vi "HMI object.vi"(4 "HMI VI path":path, 6 "Subpanel ref":refnum<vi>, 8 "error in":errorcluster, 9 "HMI cluster":T2={"Elapsed time in current state"=0.0, "smooth interval (s)"=0.0, "Process State"=1, "Current Control settings"=[]} {"Current Control settings"."fractional duty" format="%#_3g"; "smooth interval (s)" format="%.3f"; "Elapsed time in current state" format="%.2f"}, 11 "command":T4) -> (0 "error out":errorcluster, 1 "HMI Failure":bool, 3 "HMI VI ref out":T3)   [LabVIEW 2012]
uses:
  HMI command.ctl
  HMI VI type.ctl
  switch and fraction.ctl
  DAQ configuration/Sensor buffer command.ctl
  logic buffer cmd.ctl
panel:
  in  "Control names":string[](array[string])=["Current Control settings", "Sensor Data smoothed", "Set Points", "Elapsed time in current state", "Process State"]
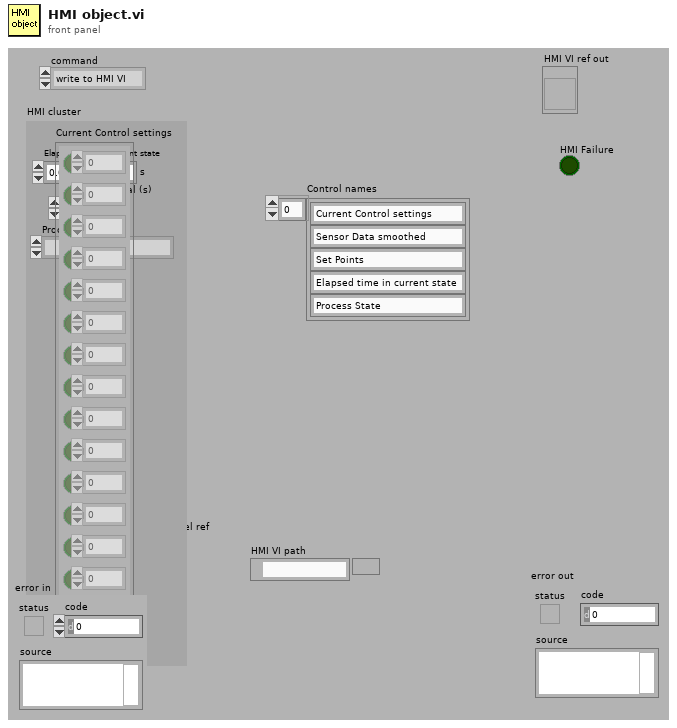
[diagram p1: front panel]
types:
  T1 = typedef "switch and fraction.ctl" = cluster{"switch":bool, "fractional duty":dbl}[]
  T2 = cluster{"Elapsed time in current state":dbl, "smooth interval (s)":sgl, "Process State":u16, "Current Control settings":T1}
  T3 = typedef "HMI VI type.ctl" = refnum<vi>
  T4 = typedef "HMI command.ctl" = enum16{"write to HMI VI", "Disconnect HMI VI", "Connect HMI VI", "Load Subpanel"}
  T5 = typedef "logic buffer cmd.ctl" = enum16{"read", "write ouput settings", "write rules", "write setpoints", "write output descriptions", "write all", "calculate setpoints", "save", "open", "Load all setpoint code", "Load one setpoint code", "Configure one setpoint code"}
  T6 = typedef "Sensor buffer command.ctl" = enum16{"read average", "read recent", "read all", "write", "configure", "clear"}
  T7 = typedef "variable setpoint.ctl" = cluster{"name":string, "unit":string, "value":dbl, "Type":enum16{"Constant", "Variable"}, "variable":cluster{"selected sensors":i32[], "selected set points":i32[], "VI":path, "Data average interval":T8, "code ref":T9}}
  T8 = typedef "data ave interval.ctl" = dbl
  T9 = typedef "type specifier for control code.ctl" = refnum<vi>
  T10 = typedef "Sensor data.ctl" = cluster{" Sensor array":T11[], "Time":dbl}
  T11 = typedef "sensor cluster.ctl" = cluster{"voltage":sgl, "scaled":sgl, "units":string, "Out of Range":bool}
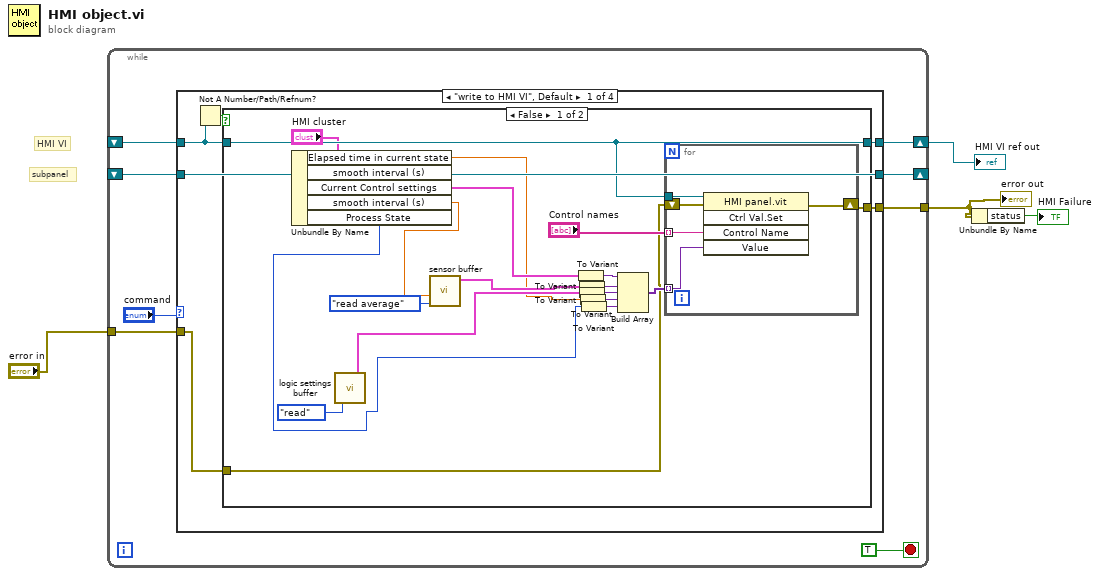
[diagram p0: block diagram]
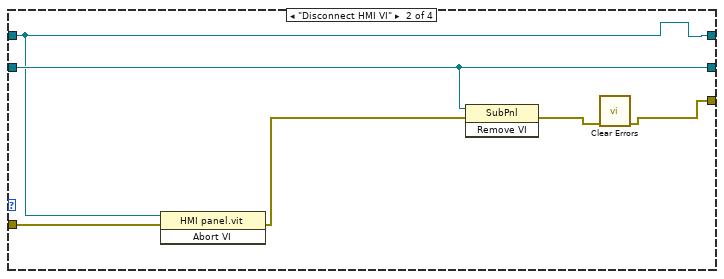
[diagram p3: hidden frame]
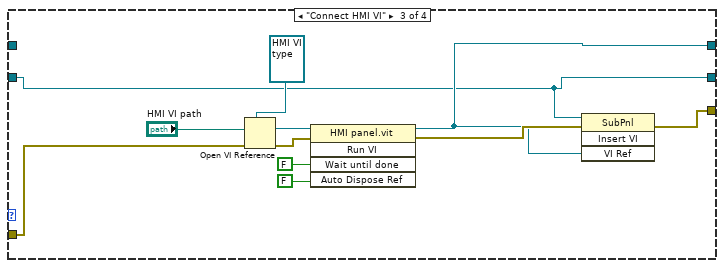
[diagram p4: hidden frame]
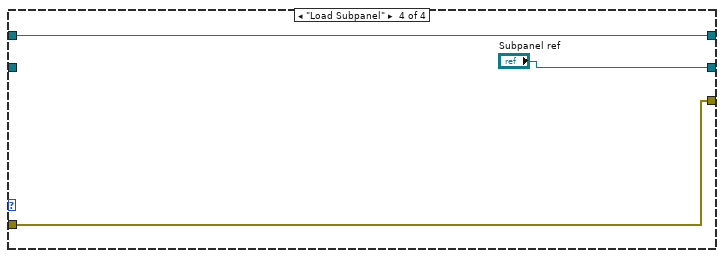
[diagram p5: hidden frame]
diagram:
  # "HMI VI"
  # "subpanel"
  n1 = while {
    tunnel: [w11] -> w4
    shift-right: [w9] -> w2
    shift-left: _ -> [w8]
    shift-right: [w7] -> _
    shift-left: _ -> [w6]
    tunnel: "error in" -> [w5]
    stop <- TRUE stop-if-true
    n2 = case shown="\"write to HMI VI\", Default" "command" {
      tunnel: [w18 w46 w55 w62] -> w11
      tunnel: w8 -> [w16 w45 _ w63]
      tunnel: [w15 w45 w56 w63] -> w9
      tunnel: w6 -> [w14 w49 w52 _]
      tunnel: [w14 w49 w52 "Subpanel ref"] -> w7
      tunnel: w5 -> [w13 w48 w51 w62]
      frame "write to HMI VI", Default {
        n3 = Not A Number/Path/Refnum?(number/path/refnum=w16) -> (NaN/Path/Refnum?=w17:bool)
        n4 = case shown="False" w17 {
          tunnel: w16 -> [w26 w44]
          tunnel: [w27 w43] -> w18
          tunnel: [w26 w44] -> w15
          tunnel: w13 -> [w20 w43]
          frame False {
            n5 = Unbundle By Name("HMI cluster") -> ("Elapsed time in current state"=w21:dbl, "Current Control settings"=w23:T1, "smooth interval (s)"=w22:sgl, "Process State"=w19:u16)  [unwired: 1 out]
            n6 = call "logic settings buffer.vi"("command"=logic_buffer_cmd."read") -> ("Set Points out"=w29:T7[])  [unwired: 11 in, 7 out]
            n7 = call "sensor buffer.vi"("command"=Sensor_buffer_command."read average", "smooth interval (s)"=w22) -> ("Sensor Data smoothed"=w31:T10)  [unwired: 3 in, 2 out]
            n8 = To Variant(anything=w23) -> (Variant=w37:variant)
            n9 = To Variant(anything=w31) -> (Variant=w36:variant)
            n10 = To Variant(anything=w29) -> (Variant=w35:variant)
            n11 = To Variant(anything=w21) -> (Variant=w34:variant)
            n12 = To Variant(anything=w19) -> (Variant=w33:variant)
            n13 = Build Array(w37, w36, w35, w34, w33) -> (w28:variant[])
            n14 = for {
              tunnel: w26 -> [w42]
              tunnel: "Control names" -> [w41] mode=indexing
              tunnel: w28 -> [w40] mode=indexing
              shift-right: [w39] -> w27
              shift-left: w20 -> [w38]
              n15 = invoke class="HMI panel.vit" method="Ctrl Val.Set"(reference=w42, error in=w38, "Control Name"=w41, "Value"=w40) -> (error out=w39:errorcluster)  [unwired: 1 in, 4 out]
            }
          }
          frame True {
          }
        }
      }
      frame "Disconnect HMI VI" {
        n16 = invoke class="HMI panel.vit" method="Abort VI"(reference=w45, error in=w48) -> (error out=w50:errorcluster)  [unwired: 1 in, 2 out]
        n17 = invoke on="Invoke Node" class="SubPnl" method="Remove VI"(reference=w49, error in=w50) -> (error out=w47:errorcluster)  [unwired: 1 in, 2 out]
        n18 = call <vilib>:"Clear Errors.vi"("error in (no error)"=w47) -> ("error out"=w46:errorcluster)  [unwired: 6 in]
      }
      frame "Connect HMI VI" {
        n19 = Open VI Reference(type specifier VI Refnum (for type only)=T3 refnum ("HMI panel"), vi path="HMI VI path", error in (no error)=w51) -> (vi reference=w57:T3, error out=w58:errorcluster)  [unwired: 3 in]
        n20 = invoke class="HMI panel.vit" method="Run VI"(reference=w57, error in=w58, "Wait until done"=FALSE, "Auto Dispose Ref"=FALSE) -> (reference out=w56:T3, error out=w59:errorcluster)  [unwired: 1 in, 3 out]
        n21 = invoke on="Invoke Node" class="SubPnl" method="Insert VI"(reference=w52, error in=w59, "VI Ref"=w56) -> (error out=w55:errorcluster)  [unwired: 1 in, 3 out]
      }
      frame "Load Subpanel" {
      }
    }
  }
  "error out" <- w4
  "HMI VI ref out" <- w2
  n22 = Unbundle By Name(w4) -> ("status"=→"HMI Failure":bool)
